vi "LS372IoscRxRyRead_DP_ver1.0.vi"(0 "GPIB ADR":i16, 3 "error in":errorcluster) -> (5 "Rx (Ohms)":dbl, 6 "dump GPIB ADR":i16, 7 "Ry (Ohms)":dbl, 9 "error out":errorcluster)   [LabVIEW 2012]
doc: "SR7265 Vos , Vx, and Vy Read out"
panel:
  out "Voltage":u16(ring) items=["2.00 uV"=1, "6.32 uV"=2, "20.0 uV"=3, "63.2 uV"=4, "200 uV"=5, "632 uV"=6, "2.0 mV"=7, "6.32 mV"=8]
  out "Current":u16(ring) items=["1.00 pA"=1, "3.16 pA"=2, "10.0 pA"=3, "31.6 pA"=4, "100 pA"=5, "316 pA"=6, "1.00 nA"=7, "3.16 nA"=8, "10 nA"=9, "31.6 nA"=10, "100 nA"=11, "316 nA"=12, "1.00 uA"=13, "3.16 uA"=14, "10.0 uA"=15, "31.6 uA"=16, "100 uA"=17, "316 uA"=18, "1.00 mA"=19, "3.16 mA"=20, "10.0 mA"=21, "31.6 mA"=22]
  out "Excitation mode":u16(ring) items=["Voltage Excitation", "Current Excitation"]
  in  "Input  Channel":u16(ring)=1 items=["All Channels", "Input 1", "Input 2", "Input 3", "Input 4", "Input 5", "Input 6", "Input 7", "Input 8"]
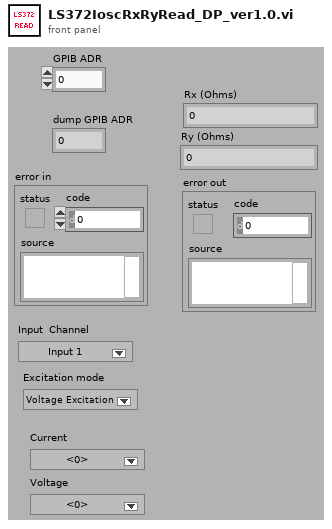
[diagram p1: front panel]
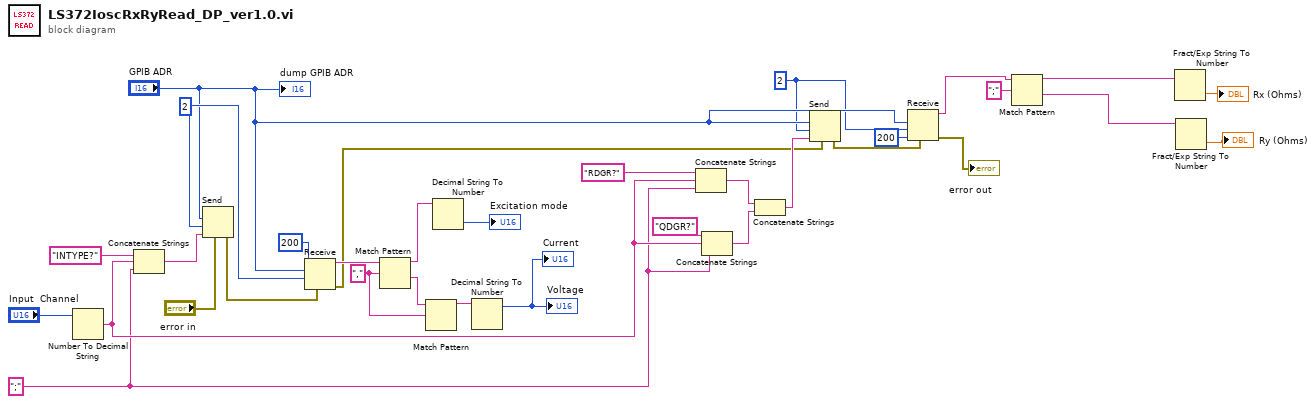
[diagram p0: block diagram]
diagram:
  w6 = i16 2 ("mode")
  w20 = "," ("regular expression")
  w13 = ";" ("string")
  w32 = i16 2 ("mode")
  n1 = Number To Decimal String(number="Input  Channel") -> (decimal integer string=w14:string)  [unwired: 1 in]
  n2 = Concatenate Strings("INTYPE?" ("data string"), w14, w13) -> (w24:string)
  n3 = Send(2:"GPIB ADR", 3:w32, 4:"error in", 5:w24) -> (8:w31:errorcluster)  [unwired: 1 in, 2 out]
  n4 = Receive(4:w31, 6:200 ("count"), 7:w32, 8:"GPIB ADR") -> (0:w9:errorcluster, 3:w23:string)  [unwired: 1 in, 2 out]
  n5 = Match Pattern(string=w23, regular expression=w20) -> (before substring=w22:string, after substring=w21:string)  [unwired: 1 in, 2 out]
  n6 = Match Pattern(string=w21, regular expression=w20) -> (before substring=w19:string)  [unwired: 1 in, 3 out]
  n7 = Decimal String To Number(string=w22) -> (number=→"Excitation mode":i32)  [unwired: 2 in, 1 out]
  n8 = Decimal String To Number(string=w19) -> (offset past number=→"Current" →"Voltage":i32)  [unwired: 2 in, 1 out]
  n9 = Concatenate Strings("RDGR?" ("data string"), w14, w13) -> (w12:string)
  n10 = Concatenate Strings("QDGR?" ("data string"), w14, w13) -> (w11:string)
  n11 = Concatenate Strings(w12, w11) -> (w10:string)
  n12 = Send(2:"GPIB ADR", 3:w6, 4:w9, 5:w10) -> (8:w8:errorcluster)  [unwired: 1 in, 2 out]
  n13 = Receive(4:w8, 6:200 ("count"), 7:w6, 8:"GPIB ADR") -> (0:→"error out":errorcluster, 3:w3:string)  [unwired: 1 in, 2 out]
  n14 = Match Pattern(string=w3, regular expression=";") -> (before substring=w2:string, after substring=w1:string)  [unwired: 1 in, 2 out]
  n15 = Fract/Exp String To Number(string=w2) -> (number=→"Rx (Ohms)":dbl)  [unwired: 3 in, 1 out]
  n16 = Fract/Exp String To Number(string=w1) -> (number=→"Ry (Ohms)":dbl)  [unwired: 3 in, 1 out]
  "dump GPIB ADR" <- "GPIB ADR"
